vi "ReaderDaemon.vi"(8 "error in (no error)":errorcluster, 10 "Variant Queue":refnum<queue>, 11 "Reader Endpoint":refnum<k21>) -> ()   [LabVIEW 2011, in "NetworkStreamReader.lvclass"]
doc: "Daemon (running in the background) which consistently checks the reader endpoint to see if a new value is available, and then passes it into the internal queue of the NetworkStreamReader if data is available."
uses:
  NetworkStreamReader.lvclass
  2-Think/2 Globals/2 Global.vi
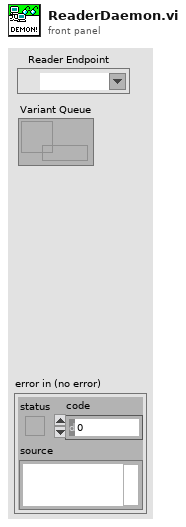
[diagram p1: front panel]
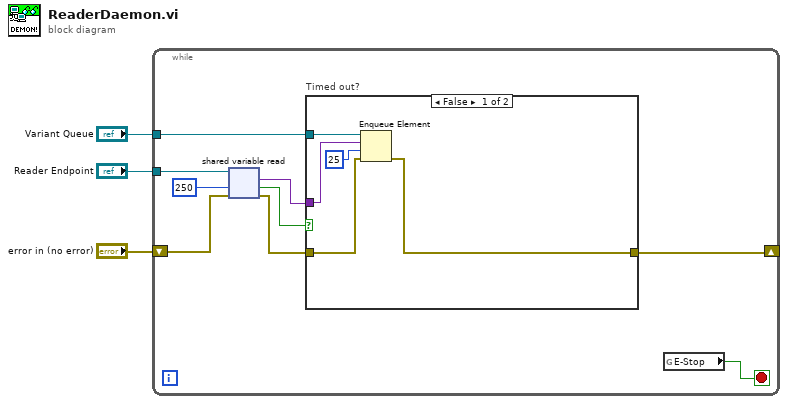
[diagram p0: block diagram]
diagram:
  n1 = while {
    tunnel: "Reader Endpoint" -> [w12]
    tunnel: "Variant Queue" -> [w6]
    shift-right: [w5] -> _
    shift-left: "error in (no error)" -> [w11]
    stop <- w4 stop-if-true
    n2 = shared-variable-read(w12, w11, 250 ("timeout in ms (-1)")) -> (w9:errorcluster, w8:bool, w7:variant)  [unwired: 1 out]
    n3 = case "Timed out?" shown="False" w8 {
      tunnel: w9 -> [w14 w18]
      tunnel: w7 -> [w16 _]
      tunnel: w6 -> [w17 _]
      tunnel: [w13 w18] -> w5
      frame False {
        n4 = Enqueue Element(queue=w17, element=w16, timeout in ms (-1)=25, error in (no error)=w14) -> (error out=w13:errorcluster)  [unwired: 2 out]
      }
      frame True {
      }
    }
    n5 = global read "2 Global.vi" "E-Stop"() -> (w4:bool)
  }
